vi "Time_Display.vi"(10 "Time Value":string, 11 "Time zone":i32=1) -> (3 "Time":string)   [LabVIEW 2019]
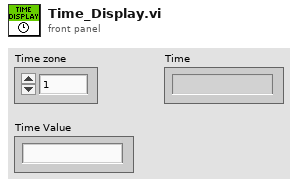
[diagram p1: front panel]
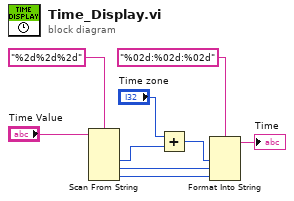
[diagram p0: block diagram]
diagram:
  n1 = Scan From String(format string="%2d%2d%2d", input string="Time Value") -> (output 1=w5:i32, output 2=w4:i32, output 3=w3:i32)  [unwired: 5 in, 3 out]
  n2 = Add(x="Time zone", y=w5) -> (x+y=w7:i32)
  n3 = Format Into String(format string="%02d:%02d:%02d", w7, w4, w3) -> (resulting string=→"Time":string)  [unwired: 2 in, 1 out]
